vi "Write_Summary_Dynamic.vi"(8 "error in":errorcluster, 9 "Sheet Name":string, 10 "Data_In":T1 {"Channel Settings"."Gain Array"."Gain 17" format="%.2f"; "Channel Settings"."Gain Array"."Gain 16" format="%.2f"; "Channel Settings"."Gain Array"."Gain 15" format="%.2f"; "Channel Settings"."Gain Array"."Gain 14" format="%.2f"; "Channel Settings"."Gain Array"."Gain 13" format="%.2f"; "Channel Settings"."Gain Array"."Gain 12" format="%.2f"; "Channel Settings"."Gain Array"."Gain 11" format="%.2f"; "Channel Settings"."Gain Array"."Gain 10" format="%.2f"; "Channel Settings"."Gain Array"."Gain 9" format="%.2f"; "Channel Settings"."Gain Array"."Gain 8" format="%.2f"; "Channel Settings"."Gain Array"."Gain 7" format="%.2f"; "Channel Settings"."Gain Array"."Gain 6" format="%.2f"; "Channel Settings"."Gain Array"."Gain 5" format="%.2f"; "Channel Settings"."Gain Array"."Gain 4" format="%.2f"; "Channel Settings"."Gain Array"."Gain 3" format="%.2f"; "Channel Settings"."Gain Array"."Gain 2" format="%.2f"; "Channel Settings"."Gain Array"."Gain 1" format="%.2f"; "Channel Settings"."Gains"."Gain 6" format="%.2f"; "Channel Settings"."Gains"."Gain 5" format="%.2f"; "Channel Settings"."Gains"."Gain 4" format="%.2f"; "Channel Settings"."Gains"."Gain 3" format="%.2f"; "Channel Settings"."Gains"."Gain 2" format="%.2f"; "Channel Settings"."Gains"."Gain 1" format="%.2f"; "Channel Settings"."User Gains"."Gain 6" format="%.2f"; "Channel Settings"."User Gains"."Gain 5" format="%.2f"; "Channel Settings"."User Gains"."Gain 4" format="%.2f"; "Channel Settings"."User Gains"."Gain 3" format="%.2f"; "Channel Settings"."User Gains"."Gain 2" format="%.2f"; "Channel Settings"."User Gains"."Gain 1" format="%.2f"; "Channel Settings"."Channel Configuration List"."Channel Configuration Cluster 17"."Current Range" items=["1 <500m>"=0.5, "2 <1>"=1.0, "5 <2.5>"=2.5, "10 <5>"=5.0, "20 <10>"=10.0, "50 <25>"=25.0]; "Channel Settings"."Channel Configuration List"."Channel Configuration Cluster 17"."Voltage Range" items=["1.5 <0.75>"=0.75, "3 <1.5>"=1.5, "6 <3>"=3.0, "10 <5>"=5.0, "15 <7.5>"=7.5, "30 <15>"=15.0, "60 <30>"=30.0, "100 <50>"=50.0, "150 <75>"=75.0, "300 <150>"=150.0, "600 <300>"=300.0, "1000 <500>"=500.0]; "Channel Settings"."Channel Configuration List"."Channel Configuration Cluster 16"."Current Range" items=["1 <500m>"=0.5, "2 <1>"=1.0, "5 <2.5>"=2.5, "10 <5>"=5.0, "20 <10>"=10.0, "50 <25>"=25.0]; "Channel Settings"."Channel Configuration List"."Channel Configuration Cluster 16"."Voltage Range" items=["1.5 <0.75>"=0.75, "3 <1.5>"=1.5, "6 <3>"=3.0, "10 <5>"=5.0, "15 <7.5>"=7.5, "30 <15>"=15.0, "60 <30>"=30.0, "100 <50>"=50.0, "150 <75>"=75.0, "300 <150>"=150.0, "600 <300>"=300.0, "1000 <500>"=500.0]; "Channel Settings"."Channel Configuration List"."Channel Configuration Cluster 15"."Current Range" items=["1 <500m>"=0.5, "2 <1>"=1.0, "5 <2.5>"=2.5, "10 <5>"=5.0, "20 <10>"=10.0, "50 <25>"=25.0]; "Channel Settings"."Channel Configuration List"."Channel Configuration Cluster 15"."Voltage Range" items=["1.5 <0.75>"=0.75, "3 <1.5>"=1.5, "6 <3>"=3.0, "10 <5>"=5.0, "15 <7.5>"=7.5, "30 <15>"=15.0, "60 <30>"=30.0, "100 <50>"=50.0, "150 <75>"=75.0, "300 <150>"=150.0, "600 <300>"=300.0, "1000 <500>"=500.0]; "Channel Settings"."Channel Configuration List"."Channel Configuration Cluster 14"."Current Range" items=["1 <500m>"=0.5, "2 <1>"=1.0, "5 <2.5>"=2.5, "10 <5>"=5.0, "20 <10>"=10.0, "50 <25>"=25.0]; "Channel Settings"."Channel Configuration List"."Channel Configuration Cluster 14"."Voltage Range" items=["1.5 <0.75>"=0.75, "3 <1.5>"=1.5, "6 <3>"=3.0, "10 <5>"=5.0, "15 <7.5>"=7.5, "30 <15>"=15.0, "60 <30>"=30.0, "100 <50>"=50.0, "150 <75>"=75.0, "300 <150>"=150.0, "600 <300>"=300.0, "1000 <500>"=500.0]; "Channel Settings"."Channel Configuration List"."Channel Configuration Cluster 13"."Current Range" items=["1 <500m>"=0.5, "2 <1>"=1.0, "5 <2.5>"=2.5, "10 <5>"=5.0, "20 <10>"=10.0, "50 <25>"=25.0]; "Channel Settings"."Channel Configuration List"."Channel Configuration Cluster 13"."Voltage Range" items=["1.5 <0.75>"=0.75, "3 <1.5>"=1.5, "6 <3>"=3.0, "10 <5>"=5.0, "15 <7.5>"=7.5, "30 <15>"=15.0, "60 <30>"=30.0, "100 <50>"=50.0, "150 <75>"=75.0, "300 <150>"=150.0, "600 <300>"=300.0, "1000 <500>"=500.0]; "Channel Settings"."Channel Configuration List"."Channel Configuration Cluster 12"."Current Range" items=["1 <500m>"=0.5, "2 <1>"=1.0, "5 <2.5>"=2.5, "10 <5>"=5.0, "20 <10>"=10.0, "50 <25>"=25.0]; "Channel Settings"."Channel Configuration List"."Channel Configuration Cluster 12"."Voltage Range" items=["1.5 <0.75>"=0.75, "3 <1.5>"=1.5, "6 <3>"=3.0, "10 <5>"=5.0, "15 <7.5>"=7.5, "30 <15>"=15.0, "60 <30>"=30.0, "100 <50>"=50.0, "150 <75>"=75.0, "300 <150>"=150.0, "600 <300>"=300.0, "1000 <500>"=500.0]; "Channel Settings"."Channel Configuration List"."Channel Configuration Cluster 11"."Current Range" items=["1 <500m>"=0.5, "2 <1>"=1.0, "5 <2.5>"=2.5, "10 <5>"=5.0, "20 <10>"=10.0, "50 <25>"=25.0]; "Channel Settings"."Channel Configuration List"."Channel Configuration Cluster 11"."Voltage Range" items=["1.5 <0.75>"=0.75, "3 <1.5>"=1.5, "6 <3>"=3.0, "10 <5>"=5.0, "15 <7.5>"=7.5, "30 <15>"=15.0, "60 <30>"=30.0, "100 <50>"=50.0, "150 <75>"=75.0, "300 <150>"=150.0, "600 <300>"=300.0, "1000 <500>"=500.0]; "Channel Settings"."Channel Configuration List"."Channel Configuration Cluster 10"."Current Range" items=["1 <500m>"=0.5, "2 <1>"=1.0, "5 <2.5>"=2.5, "10 <5>"=5.0, "20 <10>"=10.0, "50 <25>"=25.0]; "Channel Settings"."Channel Configuration List"."Channel Configuration Cluster 10"."Voltage Range" items=["1.5 <0.75>"=0.75, "3 <1.5>"=1.5, "6 <3>"=3.0, "10 <5>"=5.0, "15 <7.5>"=7.5, "30 <15>"=15.0, "60 <30>"=30.0, "100 <50>"=50.0, "150 <75>"=75.0, "300 <150>"=150.0, "600 <300>"=300.0, "1000 <500>"=500.0]; "Channel Settings"."Channel Configuration List"."Channel Configuration Cluster 9"."Voltage Range" items=["1.5 <0.75>"=0.75, "3 <1.5>"=1.5, "6 <3>"=3.0, "10 <5>"=5.0, "15 <7.5>"=7.5, "30 <15>"=15.0, "60 <30>"=30.0, "100 <50>"=50.0, "150 <75>"=75.0, "300 <150>"=150.0, "600 <300>"=300.0, "1000 <500>"=500.0]; "Channel Settings"."Channel Configuration List"."Channel Configuration Cluster 9"."Current Range" items=["10m <5m>"=0.005, "20m <10m>"=0.01, "50m <25m>"=0.025, "100m <50m>"=0.05, "200m <100m>"=0.1, "500m <250m>"=0.25, "1 <500m>"=0.5, "2 <1>"=1.0, "5 <2.5>"=2.5]; "Channel Settings"."Channel Configuration List"."Channel Configuration Cluster 8"."Voltage Range" items=["1.5 <0.75>"=0.75, "3 <1.5>"=1.5, "6 <3>"=3.0, "10 <5>"=5.0, "15 <7.5>"=7.5, "30 <15>"=15.0, "60 <30>"=30.0, "100 <50>"=50.0, "150 <75>"=75.0, "300 <150>"=150.0, "600 <300>"=300.0, "1000 <500>"=500.0]; "Channel Settings"."Channel Configuration List"."Channel Configuration Cluster 8"."Current Range" items=["10m <5m>"=0.005, "20m <10m>"=0.01, "50m <25m>"=0.025, "100m <50m>"=0.05, "200m <100m>"=0.1, "500m <250m>"=0.25, "1 <500m>"=0.5, "2 <1>"=1.0, "5 <2.5>"=2.5]; "Channel Settings"."Channel Configuration List"."Channel Configuration Cluster 7"."Voltage Range" items=["1.5 <0.75>"=0.75, "3 <1.5>"=1.5, "6 <3>"=3.0, "10 <5>"=5.0, "15 <7.5>"=7.5, "30 <15>"=15.0, "60 <30>"=30.0, "100 <50>"=50.0, "150 <75>"=75.0, "300 <150>"=150.0, "600 <300>"=300.0, "1000 <500>"=500.0]; "Channel Settings"."Channel Configuration List"."Channel Configuration Cluster 7"."Current Range" items=["10m <5m>"=0.005, "20m <10m>"=0.01, "50m <25m>"=0.025, "100m <50m>"=0.05, "200m <100m>"=0.1, "500m <250m>"=0.25, "1 <500m>"=0.5, "2 <1>"=1.0, "5 <2.5>"=2.5]; "Channel Settings"."Channel Configuration List"."Channel Configuration Cluster 6"."Voltage Range" items=["1.5 <0.75>"=0.75, "3 <1.5>"=1.5, "6 <3>"=3.0, "10 <5>"=5.0, "15 <7.5>"=7.5, "30 <15>"=15.0, "60 <30>"=30.0, "100 <50>"=50.0, "150 <75>"=75.0, "300 <150>"=150.0, "600 <300>"=300.0, "1000 <500>"=500.0]; "Channel Settings"."Channel Configuration List"."Channel Configuration Cluster 6"."Current Range" items=["10m <5m>"=0.005, "20m <10m>"=0.01, "50m <25m>"=0.025, "100m <50m>"=0.05, "200m <100m>"=0.1, "500m <250m>"=0.25, "1 <500m>"=0.5, "2 <1>"=1.0, "5 <2.5>"=2.5]; "Channel Settings"."Channel Configuration List"."Channel Configuration Cluster 5"."Voltage Range" items=["1.5 <0.75>"=0.75, "3 <1.5>"=1.5, "6 <3>"=3.0, "10 <5>"=5.0, "15 <7.5>"=7.5, "30 <15>"=15.0, "60 <30>"=30.0, "100 <50>"=50.0, "150 <75>"=75.0, "300 <150>"=150.0, "600 <300>"=300.0, "1000 <500>"=500.0]; "Channel Settings"."Channel Configuration List"."Channel Configuration Cluster 5"."Current Range" items=["10m <5m>"=0.005, "20m <10m>"=0.01, "50m <25m>"=0.025, "100m <50m>"=0.05, "200m <100m>"=0.1, "500m <250m>"=0.25, "1 <500m>"=0.5, "2 <1>"=1.0, "5 <2.5>"=2.5]; "Channel Settings"."Channel Configuration List"."Channel Configuration Cluster 4"."Voltage Range" items=["1.5 <0.75>"=0.75, "3 <1.5>"=1.5, "6 <3>"=3.0, "10 <5>"=5.0, "15 <7.5>"=7.5, "30 <15>"=15.0, "60 <30>"=30.0, "100 <50>"=50.0, "150 <75>"=75.0, "300 <150>"=150.0, "600 <300>"=300.0, "1000 <500>"=500.0]; "Channel Settings"."Channel Configuration List"."Channel Configuration Cluster 4"."Current Range" items=["10m <5m>"=0.005, "20m <10m>"=0.01, "50m <25m>"=0.025, "100m <50m>"=0.05, "200m <100m>"=0.1, "500m <250m>"=0.25, "1 <500m>"=0.5, "2 <1>"=1.0, "5 <2.5>"=2.5]; "Channel Settings"."Channel Configuration List"."Channel Configuration Cluster 3"."Voltage Range" items=["1.5 <0.75>"=0.75, "3 <1.5>"=1.5, "6 <3>"=3.0, "10 <5>"=5.0, "15 <7.5>"=7.5, "30 <15>"=15.0, "60 <30>"=30.0, "100 <50>"=50.0, "150 <75>"=75.0, "300 <150>"=150.0, "600 <300>"=300.0, "1000 <500>"=500.0]; "Channel Settings"."Channel Configuration List"."Channel Configuration Cluster 3"."Current Range" items=["10m <5m>"=0.005, "20m <10m>"=0.01, "50m <25m>"=0.025, "100m <50m>"=0.05, "200m <100m>"=0.1, "500m <250m>"=0.25, "1 <500m>"=0.5, "2 <1>"=1.0, "5 <2.5>"=2.5]; "Channel Settings"."Channel Configuration List"."Channel Configuration Cluster 2"."Voltage Range" items=["1.5 <0.75>"=0.75, "3 <1.5>"=1.5, "6 <3>"=3.0, "10 <5>"=5.0, "15 <7.5>"=7.5, "30 <15>"=15.0, "60 <30>"=30.0, "100 <50>"=50.0, "150 <75>"=75.0, "300 <150>"=150.0, "600 <300>"=300.0, "1000 <500>"=500.0]; "Channel Settings"."Channel Configuration List"."Channel Configuration Cluster 2"."Current Range" items=["10m <5m>"=0.005, "20m <10m>"=0.01, "50m <25m>"=0.025, "100m <50m>"=0.05, "200m <100m>"=0.1, "500m <250m>"=0.25, "1 <500m>"=0.5, "2 <1>"=1.0, "5 <2.5>"=2.5]; "Channel Settings"."Channel Configuration List"."Channel Configuration Cluster"."Voltage Range" items=["1.5 <0.75>"=0.75, "3 <1.5>"=1.5, "6 <3>"=3.0, "10 <5>"=5.0, "15 <7.5>"=7.5, "30 <15>"=15.0, "60 <30>"=30.0, "100 <50>"=50.0, "150 <75>"=75.0, "300 <150>"=150.0, "600 <300>"=300.0, "1000 <500>"=500.0]; "Channel Settings"."Channel Configuration List"."Channel Configuration Cluster"."Current Range" items=["10m <5m>"=0.005, "20m <10m>"=0.01, "50m <25m>"=0.025, "100m <50m>"=0.05, "200m <100m>"=0.1, "500m <250m>"=0.25, "1 <500m>"=0.5, "2 <1>"=1.0, "5 <2.5>"=2.5]; "Channel Settings"."Settling Delay" min=0.0 format="%<%H:%M:%S>t"; "Input Data 1D"."WT1800 Averages"."Vrms" format="%.3f"; "Input Data 1D"."WT1800 Averages"."Irms" format="%.3f"; "Input Data 1D"."WT1800 Averages"."Power" format="%.3f"; "Input Data 1D"."WT1800 Averages"."Vpkpk" format="%.3f"; "Input Data 1D"."WT1800 Averages"."Ipkpk" format="%.3f"; "Input Data 1D"."WT1800 Measurements"."Vrms" format="%.3f"; "Input Data 1D"."WT1800 Measurements"."Irms" format="%.3f"; "Input Data 1D"."WT1800 Measurements"."Power" format="%.3f"; "Input Data 1D"."WT1800 Measurements"."Vpkpk" format="%.3f"; "Input Data 1D"."WT1800 Measurements"."Ipkpk" format="%.3f"; "Input Data 1D"."DSA Averages"."Vrms" format="%.3f"; "Input Data 1D"."DSA Averages"."Vdc" format="%.3f"; "Input Data 1D"."DSA Averages"."Vpk+" format="%.3f"; "Input Data 1D"."DSA Averages"."Vpk-" format="%.3f"; "Input Data 1D"."DSA Averages"."Vpkpk" format="%.3f"; "Input Data 1D"."DSA Measurements"."Vrms" format="%.3f"; "Input Data 1D"."DSA Measurements"."Vdc" format="%.3f"; "Input Data 1D"."DSA Measurements"."Vpk+" format="%.3f"; "Input Data 1D"."DSA Measurements"."Vpk-" format="%.3f"; "Input Data 1D"."DSA Measurements"."Vpkpk" format="%.3f"}, 11 "NI_report in":refnum<class "NI_report.lvclass">) -> (0 "error out":errorcluster, 3 "NI_report out":refnum<class "NI_report.lvclass">)   [LabVIEW 2021]
doc: "This VI writes summary data dynamically as per the voltage steps. If voltage steps increases also, it will update the data automatically"
uses:
  Datalog Controls/Data.ctl
  <vilib>/Utility/NIReport.llb/NI_report.lvclass
  Controls/Datalog Cluster Array.ctl
  Controls/Datalog Bundle Control.ctl
  Controls/WT1800 Functions.ctl
  Controls/WT1800 Measurements.ctl
  Controls/WT1800 Readings.ctl
  Controls/DSA Functions.ctl
  Controls/DSA Measurements.ctl
  Controls/DSA Readings.ctl
  Controls/Settings Control.ctl
  Controls/Channel Configuration List.ctl
  Controls/Channel Configuration Cluster.ctl
  Controls/Channel Configuration Cluster High Current.ctl
  Controls/Gain Averages.ctl
  Controls/Gain Array.ctl
  Datalog Controls/Select_Data.ctl
  <vilib>/addons/_office/_exclsub.llb/font.ctl
  <vilib>/Utility/NIReport.llb/Append Text Table to Report (wrap).vi
  <vilib>/addons/_office/NI_ReportGenerationToolkit.lvlib
  <vilib>/Utility/NIReport.llb/Excel/NI_Excel.lvclass
  <vilib>/Utility/NIReport.llb/Append Image to Report (path wrap).vi
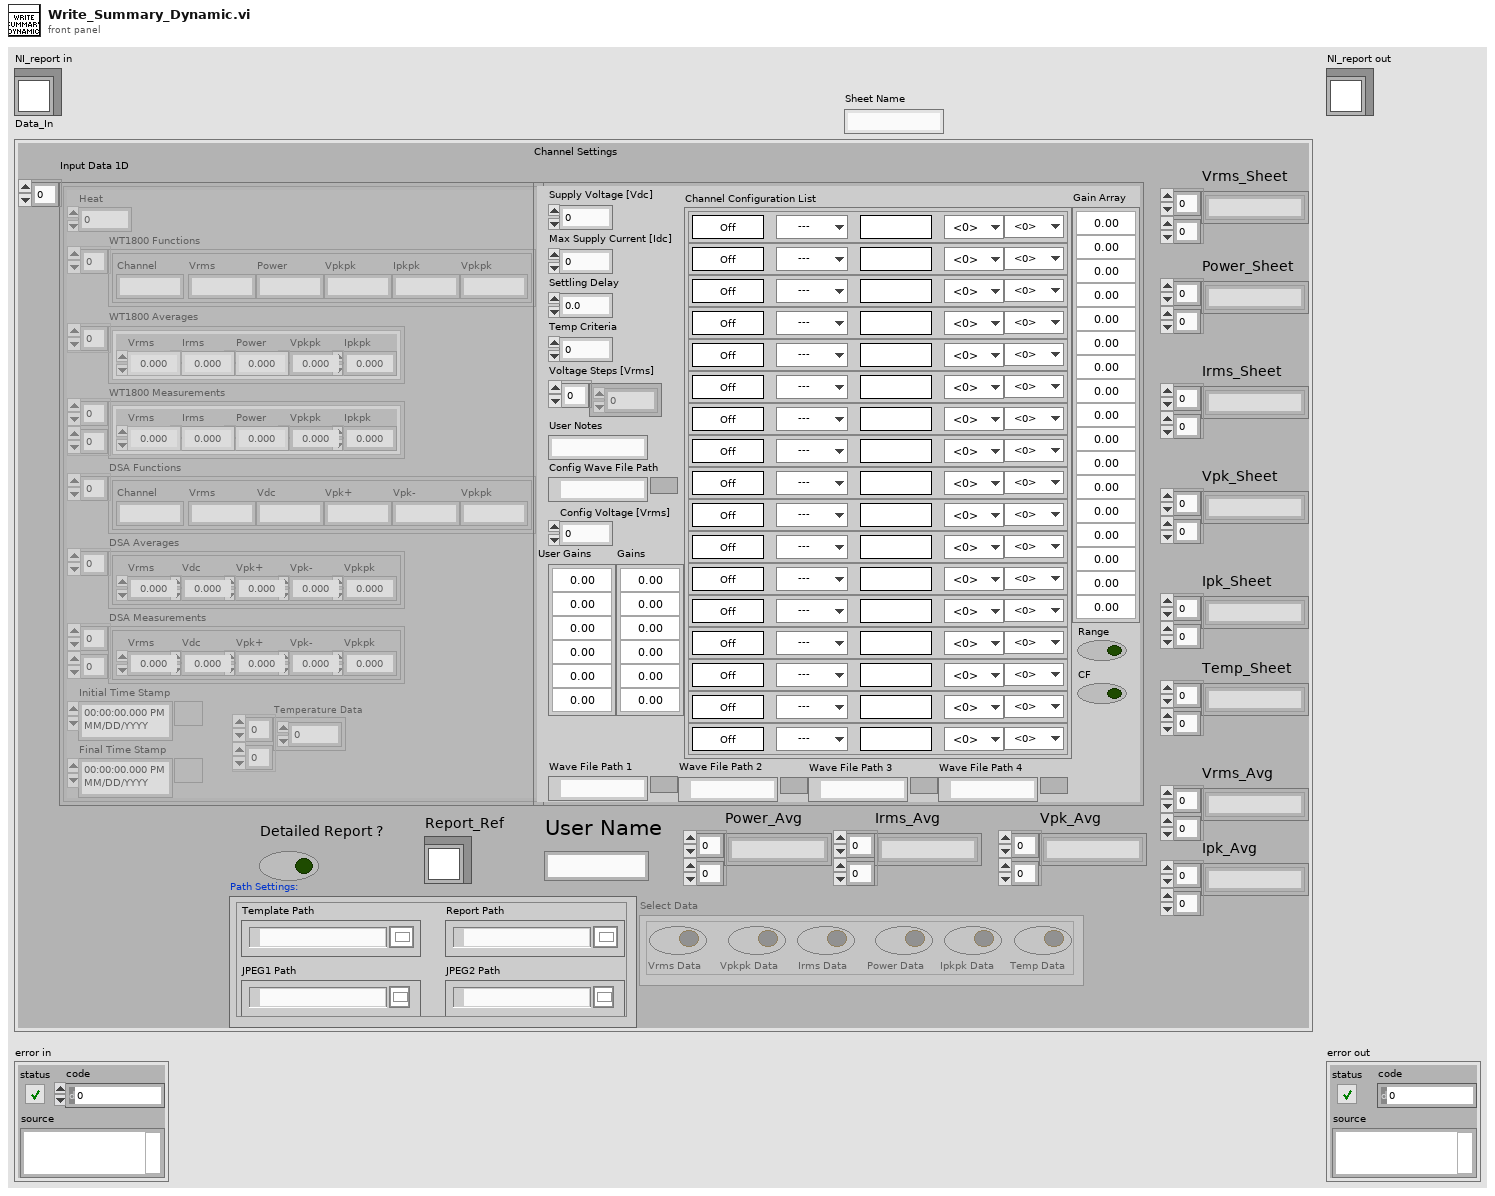
[diagram p1: front panel]
types:
  T1 = typedef "Data.ctl" = cluster{"Input Data 1D":T2, "Channel Settings":T10, "Select Data":T16, "Detailed Report ?":bool, "Path Settings:":cluster{"Template Path ":path, "Report Path":path, "JPEG1 Path ":path, "JPEG2 Path":path}, "Vrms_Sheet":string[][], "Irms_Sheet":string[][], "Power_Sheet":string[][], "Vpk_Sheet":string[][], "Ipk_Sheet":string[][], "Vrms_Avg":string[][], "Irms_Avg":string[][], "Power_Avg":string[][], "Vpk_Avg":string[][], "Ipk_Avg":string[][], "Report_Ref":refnum<class "NI_report.lvclass">, "User Name":string, "Temp_Sheet":string[][]}
  T2 = typedef "Datalog Cluster Array.ctl" = T3[]
  T3 = typedef "Datalog Bundle Control.ctl" = cluster{"Heat":dbl, "WT1800 Functions":T4, "WT1800 Averages":T5, "WT1800 Measurements":T6[][], "DSA Functions":T7, "DSA Averages":T8, "DSA Measurements":T9[][], "Initial Time Stamp":timestamp, "Final Time Stamp":timestamp, "Temperature Data":sgl[][]}
  T4 = typedef "WT1800 Functions.ctl" = cluster{"Channel":string, "Vrms":string, "Power":string, "Vpkpk":string, "Ipkpk":string, "Vpkpk":string}[]
  T5 = typedef "WT1800 Measurements.ctl" = T6[]
  T6 = typedef "WT1800 Readings.ctl" = cluster{"Vrms":sgl, "Irms":sgl, "Power":sgl, "Vpkpk":sgl, "Ipkpk":sgl}
  T7 = typedef "DSA Functions.ctl" = cluster{"Channel":string, "Vrms":string, "Vdc":string, "Vpk+":string, "Vpk-":string, "Vpkpk":string}[]
  T8 = typedef "DSA Measurements.ctl" = T9[]
  T9 = typedef "DSA Readings.ctl" = cluster{"Vrms":sgl, "Vdc":sgl, "Vpk+":sgl, "Vpk-":sgl, "Vpkpk":sgl}
  T10 = typedef "Settings Control.ctl" = cluster{"Supply Voltage [Vdc]":sgl, "Max Supply Current [Idc]":sgl, "Settling Delay":dbl, "Temp Criteria":sgl, "Voltage Steps [Vrms]":sgl[], "User Notes":string, "Config Wave File Path":path, "Config Voltage [Vrms]":sgl, "Channel Configuration List":T11, "User Gains":T14, "Gains":T14, "Gain Array":T15, "Wave File Path 1":path, "Wave File Path 2":path, "Wave File Path 3":path, "Wave File Path 4":path, "Range":bool, "CF":bool}
  T11 = typedef "Channel Configuration List.ctl" = cluster{"Channel Configuration Cluster":T12, "Channel Configuration Cluster 2":T12, "Channel Configuration Cluster 3":T12, "Channel Configuration Cluster 4":T12, "Channel Configuration Cluster 5":T12, "Channel Configuration Cluster 6":T12, "Channel Configuration Cluster 7":T12, "Channel Configuration Cluster 8":T12, "Channel Configuration Cluster 9":T12, "Channel Configuration Cluster 10":T13, "Channel Configuration Cluster 11":T13, "Channel Configuration Cluster 12":T13, "Channel Configuration Cluster 13":T13, "Channel Configuration Cluster 14":T13, "Channel Configuration Cluster 15":T13, "Channel Configuration Cluster 16":T13, "Channel Configuration Cluster 17":T13}
  T12 = typedef "Channel Configuration Cluster.ctl" = cluster{"Input":enum16{"---", "1", "1 AVG", "2", "2 AVG", "3", "3 AVG", "4", "4 AVG"}, "Enable":bool, "User Notes":string, "Voltage Range":dbl, "Current Range":dbl}
  T13 = typedef "Channel Configuration Cluster High Current.ctl" = cluster{"Input":enum16{"---", "1", "1 AVG", "2", "2 AVG", "3", "3 AVG", "4", "4 AVG"}, "Enable":bool, "User Notes":string, "Voltage Range":dbl, "Current Range":dbl}
  T14 = typedef "Gain Averages.ctl" = cluster{"Gain 1":dbl, "Gain 2":dbl, "Gain 3":dbl, "Gain 4":dbl, "Gain 5":dbl, "Gain 6":dbl}
  T15 = typedef "Gain Array.ctl" = cluster{"Gain 1":dbl, "Gain 2":dbl, "Gain 3":dbl, "Gain 4":dbl, "Gain 5":dbl, "Gain 6":dbl, "Gain 7":dbl, "Gain 8":dbl, "Gain 9":dbl, "Gain 10":dbl, "Gain 11":dbl, "Gain 12":dbl, "Gain 13":dbl, "Gain 14":dbl, "Gain 15":dbl, "Gain 16":dbl, "Gain 17":dbl}
  T16 = typedef "Select_Data.ctl" = cluster{"Vrms Data":bool, "Vpkpk Data":bool, "Irms Data":bool, "Power Data":bool, "Ipkpk Data":bool, "Temp Data":bool}
  T17 = typedef "NI_ReportGenerationToolkit.lvlib/font.ctl" = cluster{"font name":string, "font size":dbl, "bold":u16, "italic":u16, "underline":u16, "strike through":u16, "font color":u32}
  T18 = cluster{"position (excel)":cluster{"row":i32, "column":i32}, "name (excel)":string, "bookmark (word)":string}
  T19 = cluster{"on/off":bool, "weight":i32, "color":u32}
  T20 = cluster{"position (Excel)":cluster{"row":i32, "column":i32}, "name (Excel)":string, "bookmark (Word)":string}
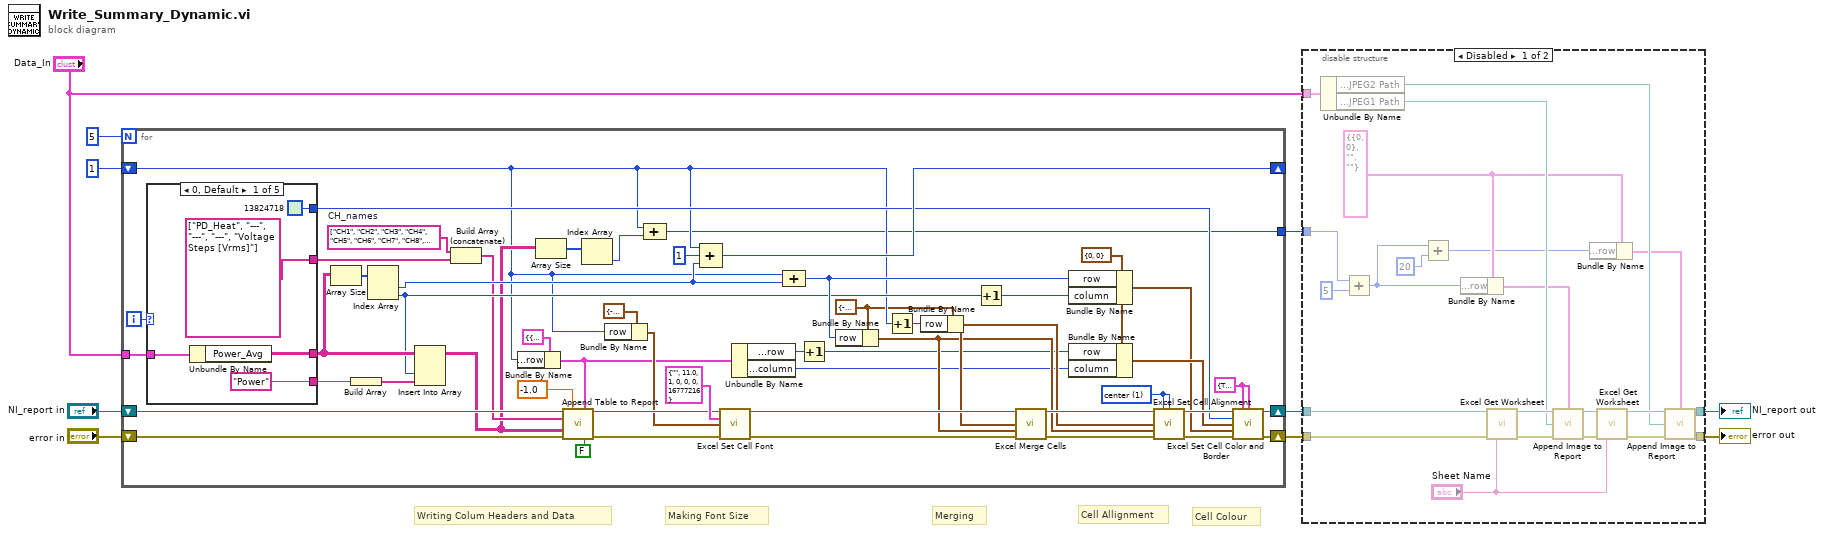
[diagram p0: block diagram]
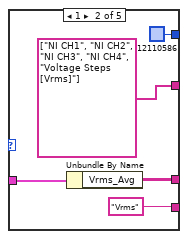
[diagram p3: hidden frame]
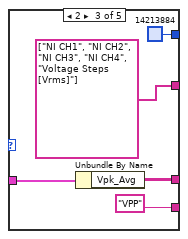
[diagram p4: hidden frame]
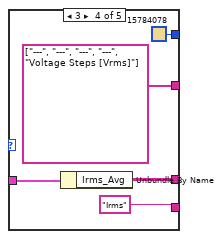
[diagram p5: hidden frame]
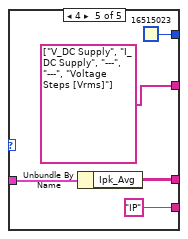
[diagram p6: hidden frame]
diagram:
  # "Cell Colour"
  # "Cell Allignment"
  # "Merging"
  # "Making Font Size"
  # "Writing Colum Headers and Data"
  n1 = for {
    N: 5 -> [_]
    shift-right: [w39] -> w6
    shift-left: "error in" -> [w62]
    shift-right: [w38] -> w5
    shift-left: "NI_report in" -> [w61]
    tunnel: "Data_In" -> [w57]
    shift-right: [w55] -> _
    shift-left: 1 ("row") -> [w14]
    tunnel: [w13] -> w1
    i -> [w60]
    w34 = T19 {"on/off"=TRUE, "weight"=2, "color"=0} ("inside border")
    w11 = cluster{"row":i32, "column":i32} {"row"=0, "column"=0} ("start (-1, -1)")
    w20 = 1 items=["top", "center", "bottom"] ("vertical alignment (top)")
    w12 = cluster{"row":i32, "column":i32} {"row"=-1, "column"=24} ("start (-1, -1)")
    w53 = string[] ["CH1", "CH2", "CH3", "CH4", "CH5", "CH6", "CH7", "CH8", "CH9", "CH10", "CH11", "CH12", "CH13", "CH14", "CH15", "CH16", "CH17", "CH18"]  # CH_names
    n2 = case shown="0, Default" w60 {
      tunnel: [w66 w71 w76 w81 w86] -> w26
      tunnel: w57 -> [w67 w72 w77 w82 w87]
      tunnel: [string[] ["PD_Heat", "---", "---", "---", "Voltage Steps [Vrms]"] ("element") string[] ["NI CH1", "NI CH2", "NI CH3", "NI CH4", "Voltage Steps [Vrms]"] ("element") string[] ["NI CH1", "NI CH2", "NI CH3", "NI CH4", "Voltage Steps [Vrms]"] ("element") string[] ["---", "---", "---", "---", "Voltage Steps [Vrms]"] ("element") string[] ["V_DC Supply", "I_DC Supply", "---", "---", "Voltage Steps [Vrms]"] ("element")] -> w52
      tunnel: [u32 13824718 ("background color (w)") u32 12110586 ("background color (w)") u32 14213884 ("background color (w)") u32 15784078 ("background color (w)") u32 16515023 ("background color (w)")] -> w37
      tunnel: ["Power" "Vrms" "VPP" "Irms" "IP"] -> w24
      frame 0, Default {
        n3 = Unbundle By Name(w67) -> ("Power_Avg"=w66:string[][])
      }
      frame 1 {
        n4 = Unbundle By Name(w72) -> ("Vrms_Avg"=w71:string[][])
      }
      frame 2 {
        n5 = Unbundle By Name(w77) -> ("Vpk_Avg"=w76:string[][])
      }
      frame 3 {
        n6 = Unbundle By Name(w82) -> ("Irms_Avg"=w81:string[][])
      }
      frame 4 {
        n7 = Unbundle By Name(w87) -> ("Ipk_Avg"=w86:string[][])
      }
    }
    n8 = Array Size(array=w26) -> (size(s)=w56:i32[])
    n9 = Build Array(w24) -> (w23:string[])
    n10 = Index Array(array=w56) -> (element #1=w21:i32, element #2=w25:i32)  [unwired: 2 in]
    n11 = Insert Into Array(array=w26, index (col)=w25, new element=w23) -> (w17:string[][])  [unwired: 1 in]
    n12 = Build Array (concatenate)(w53, w52) -> (w18:string[])
    n13 = Bundle By Name(cluster=T18 {"position (excel)"={"row"=0, "column"=1}, "name (excel)"="", "bookmark (word)"=""}, "position (excel).row"=w14) -> (w35:T18)
    n14 = Array Size(array=w17) -> (size(s)=w16:i32[])
    n15 = call-poly <vilib>:"Append Table to Report.vi"("report in"=w61, "column width (1)"=-1.0, "MS Office parameters"=w35, "column headers"=w18, "text data"=w17, "error in (no error)"=w62, "show grid lines (YES)"=FALSE) -> ("report out"=w48:refnum<class "NI_report.lvclass">, "error out"=w50:errorcluster)  [unwired: 5 in, 2 out]
    n16 = Index Array(array=w16) -> (element=w15:i32)  [unwired: 1 in]
    n17 = Bundle By Name(cluster=cluster{"row":i32, "column":i32} {"row"=-1, "column"=-1} ("start (-1, -1)"), "row"=w14) -> (w42:cluster{"row":i32, "column":i32})
    n18 = Compound Arithmetic op=ADD(w14, w15) -> (w13:i32)
    n19 = Compound Arithmetic op=ADD(w14, 1 ("value"), w21) -> (w55:i32)
    n20 = call <vilib>:"Excel Set Cell Font.vi"("report in"=w48, "font"=T17 {"font name"="", "font size"=11.0, "bold"=1, "italic"=0, "underline"=0, "strike through"=0, "font color"=16777216}, "start (-1, -1)"=w42, "error in (no error)"=w50) -> ("report out"=w46:refnum<class "NI_report.lvclass">, "error out"=w47:errorcluster)  [unwired: 10 in]
    n21 = Unbundle By Name(w35) -> ("position (excel).row"=w33:i32, "position (excel).column"=w31:i32)
    n22 = Compound Arithmetic op=ADD(w14, w21) -> (w27:i32)
    n23 = Increment(x=w33) -> (x+1=w32:i32)
    n24 = Bundle By Name(cluster=w12, "row"=w27) -> (w36:cluster{"row":i32, "column":i32})
    n25 = Increment(x=w14) -> (x+1=w29:i32)
    n26 = Bundle By Name(cluster=w12, "row"=w29) -> (w43:cluster{"row":i32, "column":i32})
    n27 = Increment(x=w25) -> (x+1=w28:i32)
    n28 = call <vilib>:"Excel Merge Cells.vi"("report in"=w46, "start (-1, -1)"=w43, "end (-1, -1)"=w36, "error in (no error)"=w47) -> ("report out"=w44:refnum<class "NI_report.lvclass">, "error out"=w45:errorcluster)  [unwired: 10 in]
    n29 = Bundle By Name(cluster=w11, "row"=w27, "column"=w28) -> (w19:cluster{"row":i32, "column":i32})
    n30 = Bundle By Name(cluster=w11, "row"=w32, "column"=w31) -> (w30:cluster{"row":i32, "column":i32})
    n31 = call <vilib>:"Excel Set Cell Alignment.vi"("report in"=w44, "vertical alignment (top)"=w20, "horizontal alignment (left)"=w20, "start (-1, -1)"=w43, "end (-1, -1)"=w36, "error in (no error)"=w45) -> ("report out"=w40:refnum<class "NI_report.lvclass">, "error out"=w41:errorcluster)  [unwired: 8 in]
    n32 = call <vilib>:"Excel Set Cell Color and Border.vi"("report in"=w40, "inside border"=w34, "outside border"=w34, "background color (w)"=w37, "start (-1, -1)"=w30, "end (-1, -1)"=w19, "error in (no error)"=w41) -> ("report out"=w38:refnum<class "NI_report.lvclass">, "error out"=w39:errorcluster)  [unwired: 7 in]
  }
  n33 = disable-structure shown="Disabled" {
    disable-tunnel: w6 -> [w101 w110]
    disable-tunnel: w5 -> [w100 w111]
    disable-tunnel: "Data_In" -> [w99 _]
    disable-tunnel: [w92 w111] -> w3
    disable-tunnel: [w91 w110] -> w2
    disable-tunnel: w1 -> [w89 _]
    frame Disabled {
      w96 = T20 {"position (Excel)"={"row"=0, "column"=0}, "name (Excel)"="", "bookmark (Word)"=""} ("MS Office parameters")
      n34 = Unbundle By Name(w99) -> ("Path Settings:.JPEG2 Path"=w102:path, "Path Settings:.JPEG1 Path"=w103:path)
      n35 = Add(x=w89, y=5) -> (x+y=w88:i32)
      n36 = Add(x=w88, y=20) -> (x+y=w93:i32)
      n37 = Bundle By Name(cluster=w96, "position (Excel).row"=w88) -> (w97:T20)
      n38 = call <vilib>:"Excel Get Worksheet.vi"("report in"=w100, "error in (no error)"=w101, "name (\"\")"="Sheet Name") -> ("report out"=w108:refnum<class "NI_report.lvclass">, "error out"=w109:errorcluster)  [unwired: 11 in]
      n39 = call-poly <vilib>:"Append Image to Report.vi"("report in"=w108, "MS Office parameters"=w97, "path or URL of image"=w103, "error in (no error)"=w109) -> ("report out"=w104:refnum<class "NI_report.lvclass">, "error out"=w105:errorcluster)  [unwired: 8 in, 2 out]
      n40 = Bundle By Name(cluster=w96, "position (Excel).row"=w93) -> (w95:T20)
      n41 = call <vilib>:"Excel Get Worksheet.vi"("report in"=w104, "error in (no error)"=w105, "name (\"\")"="Sheet Name") -> ("report out"=w107:refnum<class "NI_report.lvclass">, "error out"=w106:errorcluster)  [unwired: 11 in]
      n42 = call-poly <vilib>:"Append Image to Report.vi"("report in"=w107, "MS Office parameters"=w95, "path or URL of image"=w102, "error in (no error)"=w106) -> ("report out"=w92:refnum<class "NI_report.lvclass">, "error out"=w91:errorcluster)  [unwired: 8 in, 2 out]
    }
    frame Enabled {
    }
  }
  "NI_report out" <- w3
  "error out" <- w2
